vi "Simulation.vi"() -> ()   [LabVIEW 2013]
uses:
  <vilib>/Platform/TimedLoop/XDataNode/timing_clust.ctl
  <vilib>/Platform/TimedLoop/XDataNode/nitl_modes.ctl
  <vilib>/Platform/TimedLoop/XDataNode/wakeup.ctl
  <vilib>/Analysis/coordinate.llb/Angle Units.ctl
  <vilib>/Analysis/coordinate.llb/Angle Range (Degree).ctl
  <vilib>/Analysis/coordinate.llb/Wrap Angle (scalar).vi
  <vilib>/Utility/inputDevices.llb/closeJoystick.vi
  <vilib>/Utility/inputDevices.llb/joystickAcquire.vi
  <vilib>/Platform/TimedLoop/XDataNode/XDataNode.xnode
  <vilib>/Platform/TimedLoop/XDataNode/XDNodeRunTimeDep.lvlib
  Helper Functions/ProcessorHelperFunctions.lvlib
  <vilib>/Analysis/NI_AAL_Angle.lvlib
panel:
  in  "PID Gains":cluster{"P":dbl, "I":dbl, "D":dbl}={"P"=1.0, "I"=0.0, "D"=0.0}
  in  "Error Correction Speed":dbl=0.03
  out "Wheel Pos/Speed":picture
  out "Simulation Wheel Angles":dbl[](array[numeric])
  in  "Manual Motor Control":bool=TRUE
  in  "Motor Number":u8
  out "T1":dbl
  out "T3":dbl
  out "T2":dbl
  out "T4":dbl
  out "Wheel Target Angles":dbl[](array[numeric])
  out "Motor Output Values":u16[](array[slide]) scale=0.0..512.0
  out "Status LED":bool
  in  "stop":bool
  in  "ESTOP":bool
  out "TX Data":T1
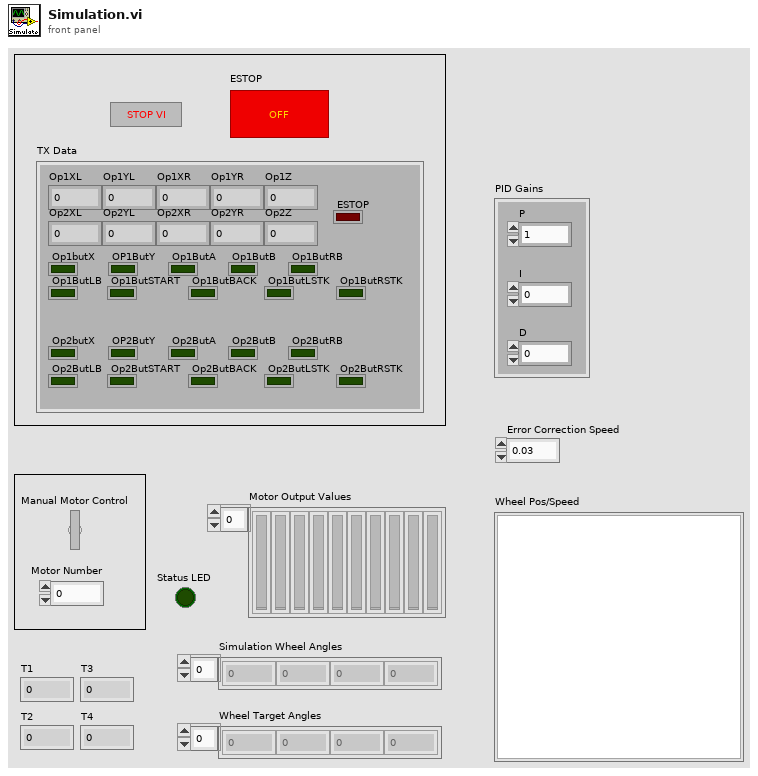
[diagram p1: front panel]
types:
  T1 = cluster{"Op2ButLSTK":bool, "Op2ButRSTK":bool, "Op1ButLSTK":bool, "Op1ButRSTK":bool, "Op1XL":i32, "Op1YL":i32, "Op1XR":i32, "Op1YR":i32, "Op1Z":i32, "Op2XL":i32, "Op2YL":i32, "Op2XR":i32, "Op2YR":i32, "Op2Z":i32, "ESTOP":bool, "Op1butX":bool, "OP1ButY":bool, "Op1ButA":bool, "Op1ButB":bool, "Op1ButRB":bool, "Op1ButLB":bool, "Op2butX":bool, "OP2ButY":bool, "Op2ButA":bool, "Op2ButB":bool, "Op2ButRB":bool, "Op2ButLB":bool, "Op2ButSTART":bool, "Op2ButBACK":bool, "Op1ButSTART":bool, "Op1ButBACK":bool}
  T2 = typedef "XDNodeRunTimeDep.lvlib/timing_clust.ctl" = cluster{"Expected End [f-1]":u64, "Actual End [f-1]":u64, "Finished Late? [f-1]":bool, "Expected End [i-1]":u64, "Actual End [i-1]":u64, "Finished Late? [i-1]":bool, "Expected Start [i]":u64, "Actual Start [i]":u64, "Expected Start [f]":u64, "Actual Start [f]":u64, "Source Name":string, "Structure Name":string, "Period":i64, "Deadline":i64, "Offset":i64, "Start":i64, "Priority":i32, "Timeout":i32, "Mode":T3, "Wakeup Reason":T4, "Error":errorcluster, "Source Type":string, "Secondary Source Type":string, "Global End Time":u64, "Global Start Time":u64, "Frame Duration":u64, "Iteration Duration":u64, "Assigned CPU":i32, "I/O Scan Engine Mode":u32}
  T3 = typedef "XDNodeRunTimeDep.lvlib/nitl_modes.ctl" = enum32{"No Change", "Process missed periods, maintain original phase", "Discard missed periods, maintain original phase", "Process missed periods, ignore original phase", "Discard missed periods, ignore original phase"}
  T4 = typedef "XDNodeRunTimeDep.lvlib/wakeup.ctl" = enum32{"Normal", "Aborted", "Asynchronous wakeup", "Timing source error", "Timed loop error", "Timeout"}
  T5 = typedef "NI_AAL_Angle.lvlib/Angle Range (Degree).ctl" = u16
  T6 = typedef "NI_AAL_Angle.lvlib/Angle Units.ctl" = i32
  T7 = cluster{"[0]":u16, "[1]":u16, "[2]":u16, "[3]":u16}
  T8 = cluster{"[0]":dbl, "[1]":dbl, "[2]":dbl, "[3]":dbl, "[4]":dbl, "[5]":dbl, "[6]":dbl, "[7]":dbl, "[8]":dbl}
  T9 = cluster{"Target Angles[0]":dbl, "Target Angles[1]":dbl, "Target Angles[2]":dbl, "Target Angles[3]":dbl}
  T10 = cluster{"X axis":i32, "Y axis":i32, "Z axis":i32, "X axis rotation":i32, "Y axis rotation":i32, "Z axis rotation":i32, "U axis":i32, "V axis":i32}
  T11 = cluster{"button 1":bool, "button 2":bool, "button 3":bool, "button 4":bool, "button 5":bool, "button 6":bool, "button 7":bool, "button 8":bool, "button 9":bool, "button 10":bool, "button 11":bool, "button 12":bool, "button 13":bool, "button 14":bool, "button 15":bool, "button 16":bool, "button 17":bool, "button 18":bool, "button 19":bool, "button 20":bool, "button 21":bool, "button 22":bool, "button 23":bool, "button 24":bool, "button 25":bool, "button 26":bool, "button 27":bool, "button 28":bool, "button 29":bool, "button 30":bool, "button 31":bool, "button 32":bool}
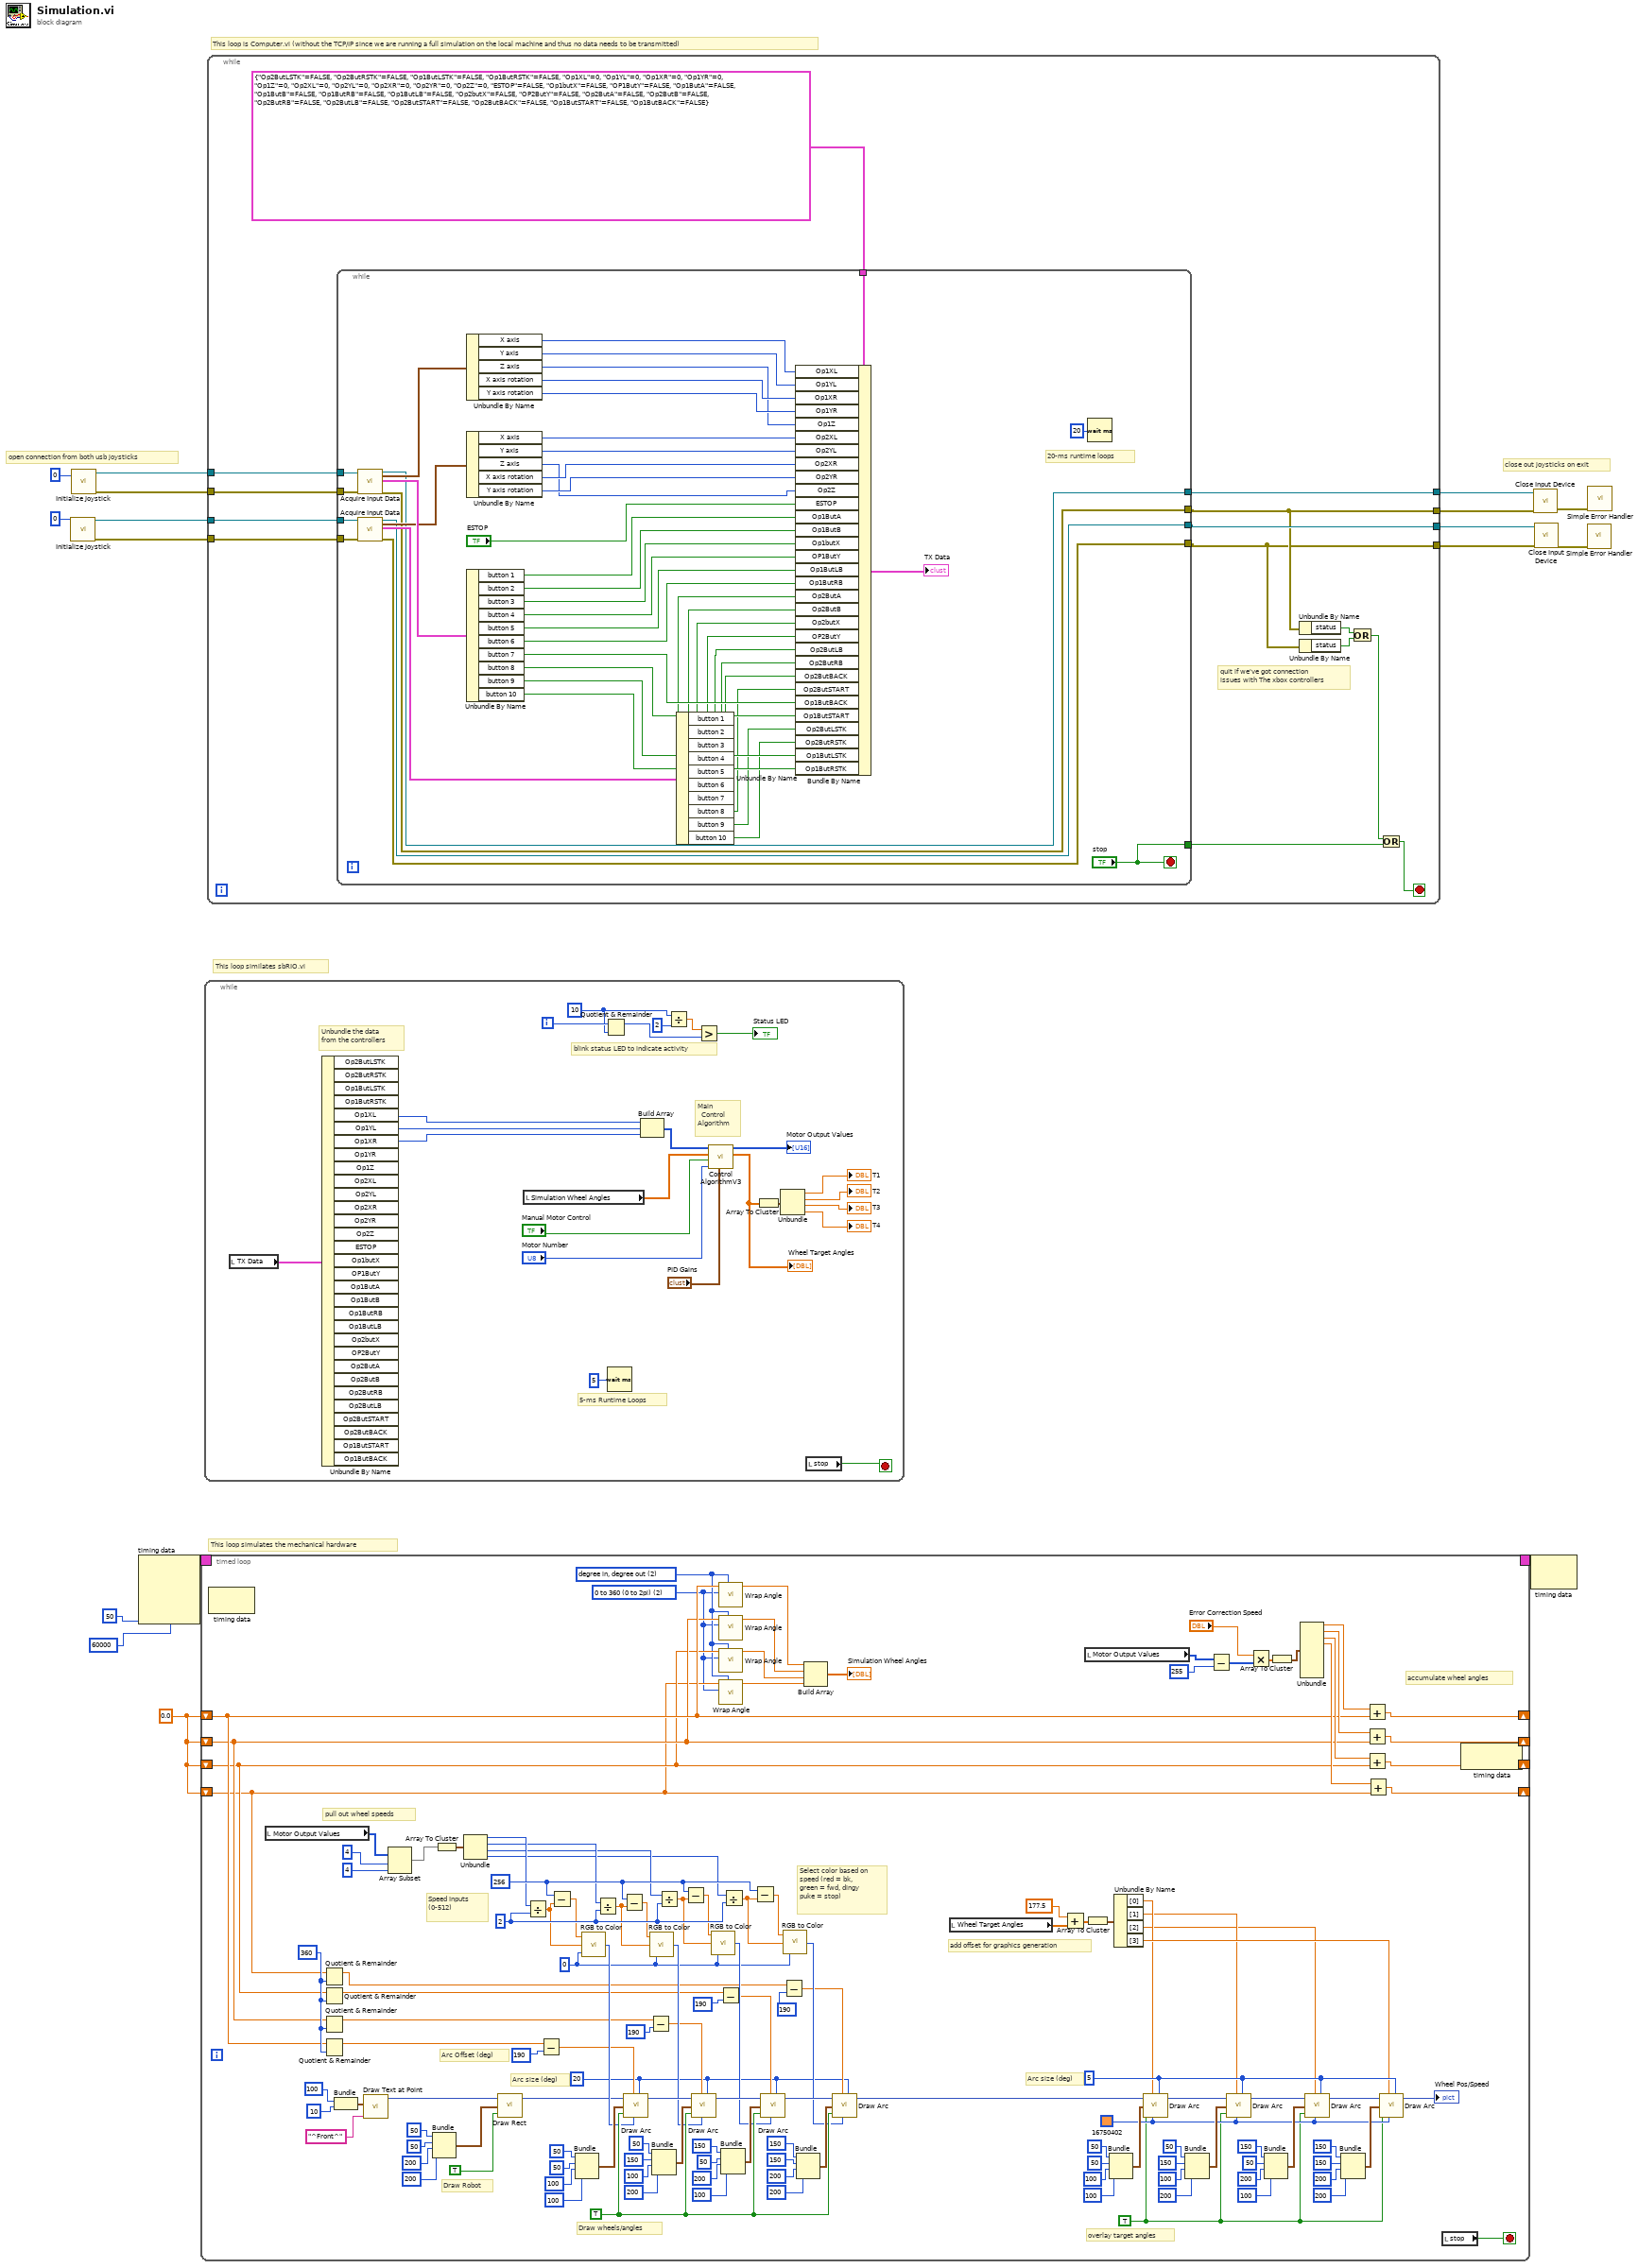
[diagram p0: block diagram]
diagram:
  w1 = 0.0
  # "This loop simulates the mechanical hardware"
  # "This loop similates sbRIO.vi"
  # "This loop is Computer.vi (without the TCP/IP since we are running a full simulation on the local machine and thus no data needs to be transmitted)"
  # "open connection from both usb joysticks"
  # "close out joysticks on exit"
  n1 = call <vilib>:"Initialize Joystick.vi"("device index"=0) -> ("error out"=w6:errorcluster, "device ID"=w7:refnum<k1>)  [unwired: 9 in]
  n2 = call <vilib>:"Initialize Joystick.vi"("device index"=0) -> ("error out"=w8:errorcluster, "device ID"=w9:refnum<k1>)  [unwired: 9 in]
  n3 = node-c288(50, 60000) -> (w5:T2)  [unwired: 2 in]
  n4 = timed-loop {
    timing: w5 -> [_]
    timing-out: [_] -> w4
    shift-right: [w148] -> _
    shift-left: w1 -> [w26]
    shift-right: [w147] -> _
    shift-left: w1 -> [w25]
    shift-right: [w149] -> _
    shift-left: w1 -> [w27]
    shift-right: [w150] -> _
    shift-left: w1 -> [w28]
    stop <- w31 stop-if-true
    w18 = T5 2 items=["none", "-180 to 180 (-pi to pi)", "0 to 360 (0 to 2pi)"] ("angle range")
    w19 = T6 2 items=["radian in, radian out", "radian in, degree out", "degree in, degree out", "degree in, radian out"] ("angle units")
    w33 = 360
    w53 = TRUE
    w56 = 5
    w57 = u32 16750402
    w87 = 20
    w32 = 0
    w104 = 2
    w105 = 256
    w117 = TRUE
    # "add offset for graphics generation"
    # "pull out wheel speeds"
    # "Arc size (deg)"
    # "overlay target angles"
    # "Arc Offset (deg)"
    # "Arc size (deg)"
    # "Speed Inputs (0-512)"
    # "Draw wheels/angles"
    # "Select color based on speed (red = bk, green = fwd, dingy puke = stop)"
    # "Draw Robot"
    # "accumulate wheel angles"
    n5 = node-c288() -> ()  [unwired: 1 in, 1 out]
    n6 = local read "Motor Output Values"() -> (w44:u16[])
    n7 = Quotient & Remainder(x=w25, y=w33) -> (x-y*floor(x/y)=w37:dbl)  [unwired: 1 out]
    n8 = Quotient & Remainder(x=w26, y=w33) -> (x-y*floor(x/y)=w36:dbl)  [unwired: 1 out]
    n9 = Quotient & Remainder(x=w27, y=w33) -> (x-y*floor(x/y)=w35:dbl)  [unwired: 1 out]
    n10 = Quotient & Remainder(x=w28, y=w33) -> (x-y*floor(x/y)=w34:dbl)  [unwired: 1 out]
    n11 = Bundle(100, 10) -> (w82:cluster{i32, i32})  [unwired: 1 in]
    n12 = call <vilib>:"Draw Text at Point.vi"("text"="^Front^", "origin"=w82) -> ("new picture"=w86:picture)  [unwired: 8 in, 1 out]
    n13 = Array Subset(array=w44, index=4, length=4) -> (w49:u16[])
    n14 = Bundle(50, 50, 200, 200) -> (w108:cluster{i32, i32, i32, i32})  [unwired: 1 in]
    n15 = Array To Cluster(array=w49) -> (cluster=w50:T7)
    n16 = Unbundle(w50) -> ("[0]"=w48:u16, "[1]"=w47:u16, "[2]"=w46:u16, "[3]"=w45:u16)
    n17 = call <vilib>:"Draw Rect.vi"("picture"=w86, "rect"=w108, "fill?(F)"=TRUE) -> ("new picture"=w106:picture)  [unwired: 6 in]
    n18 = Divide(x=w48, y=w104) -> (x/y=w103:dbl)
    n19 = Subtract(x=w34, y=190) -> (x-y=w94:dbl)
    n20 = Subtract(x=w105, y=w103) -> (x-y=w100:dbl)
    n21 = Bundle(50, 50, 100, 100) -> (w134:cluster{i32, i32, i32, i32})  [unwired: 1 in]
    n22 = call <vilib>:"RGB to Color.vi"("B"=w32, "G"=w103, "R"=w100) -> ("Color"=w116:u32)
    n23 = Divide(x=w47, y=w104) -> (x/y=w102:dbl)
    n24 = Subtract(x=w105, y=w102) -> (x-y=w99:dbl)
    n25 = call <vilib>:"Draw Arc.vi"("picture"=w106, "start angle[degrees]"=w94, "rect"=w134, "fill?(F)"=w117, "color(black)"=w116, "arc size[degrees]"=w87) -> ("new picture"=w140:picture)  [unwired: 3 in]
    n26 = Subtract(x=w35, y=190) -> (x-y=w90:dbl)
    n27 = call <vilib>:"RGB to Color.vi"("B"=w32, "G"=w102, "R"=w99) -> ("Color"=w115:u32)
    n28 = Bundle(50, 150, 100, 200) -> (w120:cluster{i32, i32, i32, i32})  [unwired: 1 in]
    n29 = Divide(x=w46, y=w104) -> (x/y=w98:dbl)
    n30 = Subtract(x=w105, y=w98) -> (x-y=w97:dbl)
    n31 = call <vilib>:"Draw Arc.vi"("picture"=w140, "start angle[degrees]"=w90, "rect"=w120, "fill?(F)"=w117, "color(black)"=w115, "arc size[degrees]"=w87) -> ("new picture"=w139:picture)  [unwired: 3 in]
    n32 = call <vilib>:"RGB to Color.vi"("B"=w32, "G"=w98, "R"=w97) -> ("Color"=w114:u32)
    n33 = call-poly <vilib>:"Wrap Angle.vi"("angle units"=w19, "angle range"=w18, "angle in"=w28) -> ("angle out"=w24:dbl)  [unwired: 7 in, 1 out]
    n34 = call-poly <vilib>:"Wrap Angle.vi"("angle units"=w19, "angle range"=w18, "angle in"=w27) -> ("angle out"=w23:dbl)  [unwired: 7 in, 1 out]
    n35 = call-poly <vilib>:"Wrap Angle.vi"("angle units"=w19, "angle range"=w18, "angle in"=w26) -> ("angle out"=w22:dbl)  [unwired: 7 in, 1 out]
    n36 = call-poly <vilib>:"Wrap Angle.vi"("angle units"=w19, "angle range"=w18, "angle in"=w25) -> ("angle out"=w21:dbl)  [unwired: 7 in, 1 out]
    n37 = Subtract(x=w36, y=190) -> (x-y=w89:dbl)
    n38 = Bundle(150, 50, 200, 100) -> (w119:cluster{i32, i32, i32, i32})  [unwired: 1 in]
    n39 = Divide(x=w45, y=w104) -> (x/y=w101:dbl)
    n40 = Subtract(x=w105, y=w101) -> (x-y=w96:dbl)
    n41 = call <vilib>:"Draw Arc.vi"("picture"=w139, "start angle[degrees]"=w89, "rect"=w119, "fill?(F)"=w117, "color(black)"=w114, "arc size[degrees]"=w87) -> ("new picture"=w138:picture)  [unwired: 3 in]
    n42 = Subtract(x=w37, y=190) -> (x-y=w88:dbl)
    n43 = call <vilib>:"RGB to Color.vi"("B"=w32, "G"=w101, "R"=w96) -> ("Color"=w113:u32)
    n44 = Bundle(150, 150, 200, 200) -> (w118:cluster{i32, i32, i32, i32})  [unwired: 1 in]
    n45 = Build Array(w24, w23, w22, w21) -> (→"Simulation Wheel Angles":dbl[])
    n46 = call <vilib>:"Draw Arc.vi"("picture"=w138, "start angle[degrees]"=w88, "rect"=w118, "fill?(F)"=w117, "color(black)"=w113, "arc size[degrees]"=w87) -> ("new picture"=w81:picture)  [unwired: 3 in]
    n47 = local read "Wheel Target Angles"() -> (w43:dbl[])
    n48 = Add(x=177.5, y=w43) -> (x+y=w42:dbl[])
    n49 = local read "Motor Output Values"() -> (w29:u16[])
    n50 = Array To Cluster(array=w42) -> (cluster=w55:T8)
    n51 = Bundle(50, 50, 100, 100) -> (w75:cluster{i32, i32, i32, i32})  [unwired: 1 in]
    n52 = Unbundle By Name(w55) -> ("[0]"=w40:dbl, "[1]"=w39:dbl, "[2]"=w38:dbl, "[3]"=w54:dbl)
    n53 = call <vilib>:"Draw Arc.vi"("picture"=w81, "start angle[degrees]"=w40, "rect"=w75, "fill?(F)"=w53, "color(black)"=w57, "arc size[degrees]"=w56) -> ("new picture"=w80:picture)  [unwired: 3 in]
    n54 = Bundle(50, 150, 100, 200) -> (w69:cluster{i32, i32, i32, i32})  [unwired: 1 in]
    n55 = Subtract(x=w29, y=255) -> (x-y=w152:i32[])
    n56 = call <vilib>:"Draw Arc.vi"("picture"=w80, "start angle[degrees]"=w39, "rect"=w69, "fill?(F)"=w53, "color(black)"=w57, "arc size[degrees]"=w56) -> ("new picture"=w63:picture)  [unwired: 3 in]
    n57 = Multiply(x="Error Correction Speed", y=w152) -> (x*y=w146:dbl[])
    n58 = Bundle(150, 50, 200, 100) -> (w64:cluster{i32, i32, i32, i32})  [unwired: 1 in]
    n59 = Array To Cluster(array=w146) -> (cluster=w151:T8)
    n60 = Unbundle(w151) -> ("[0]"=w144:dbl, "[1]"=w143:dbl, "[2]"=w142:dbl, "[3]"=w141:dbl)  [unwired: 5 out]
    n61 = call <vilib>:"Draw Arc.vi"("picture"=w63, "start angle[degrees]"=w38, "rect"=w64, "fill?(F)"=w53, "color(black)"=w57, "arc size[degrees]"=w56) -> ("new picture"=w79:picture)  [unwired: 3 in]
    n62 = Bundle(150, 150, 200, 200) -> (w58:cluster{i32, i32, i32, i32})  [unwired: 1 in]
    n63 = Add(x=w144, y=w28) -> (x+y=w150:dbl)
    n64 = Add(x=w143, y=w27) -> (x+y=w149:dbl)
    n65 = Add(x=w142, y=w26) -> (x+y=w148:dbl)
    n66 = Add(x=w141, y=w25) -> (x+y=w147:dbl)
    n67 = call <vilib>:"Draw Arc.vi"("picture"=w79, "start angle[degrees]"=w54, "rect"=w58, "fill?(F)"=w53, "color(black)"=w57, "arc size[degrees]"=w56) -> ("new picture"=→"Wheel Pos/Speed":picture)  [unwired: 3 in]
    n68 = local read "stop"() -> (w31:bool)
    n69 = node-c288() -> ()  [unwired: 1 in, 1 out]
  }
  n70 = while {
    i -> [w178]
    stop <- w163 stop-if-true
    w174 = 10
    # "Unbundle the data\nfrom the controllers"
    # "Main\n  Control\nAlgorithm"
    # "blink status LED to indicate activity"
    # "5-ms Runtime Loops"
    n71 = local read "TX Data"() -> (w165:T1)
    n72 = Unbundle By Name(w165) -> ("Op1XL"=w168:i32, "Op1YL"=w167:i32, "Op1XR"=w166:i32)  [unwired: 28 out]
    n73 = local read "Simulation Wheel Angles"() -> (w161:dbl[])
    n74 = Quotient & Remainder(x=w178, y=w174) -> (x-y*floor(x/y)=w176:i32)  [unwired: 1 out]
    n75 = Wait (ms)(milliseconds to wait=u32 5) -> ()  [unwired: 1 out]
    n76 = Build Array(w168, w167, w166) -> (w162:i32[])
    n77 = Divide(x=w174, y=2) -> (x/y=w175:dbl)
    n78 = Greater?(x=w175, y=w176) -> (0:→"Status LED":bool)
    n79 = call "Control AlgorithmV3.vi"("PID Gains"="PID Gains", "Motor to Control"="Motor Number", "Manual Control"="Manual Motor Control", "Wheel Angles"=w161, "JoystickIn"=w162) -> ("Target Angles"=w157:dbl[], "MotorsOut"=→"Motor Output Values":u16[])  [unwired: 5 in]
    "Wheel Target Angles" <- w157
    n80 = Array To Cluster(array=w157) -> (cluster=w173:T9)
    n81 = Unbundle(w173) -> ("Target Angles[0]"=→"T1":dbl, "Target Angles[1]"=→"T2":dbl, "Target Angles[2]"=→"T3":dbl, "Target Angles[3]"=→"T4":dbl)
    n82 = local read "stop"() -> (w163:bool)
  }
  n83 = while {
    tunnel: [w192] -> w15
    tunnel: [w190] -> w14
    tunnel: [w191] -> w13
    tunnel: [w189] -> w12
    tunnel: w9 -> [w185]
    tunnel: w8 -> [w184]
    tunnel: w7 -> [w183]
    tunnel: w6 -> [w182]
    stop <- w186 stop-if-true
    # "quit if we've got connection \nissues with The xbox controllers"
    n84 = while {
      tunnel: w185 -> [w239]
      tunnel: w184 -> [w238]
      tunnel: T1 {"Op2ButLSTK"=FALSE, "Op2ButRSTK"=FALSE, "Op1ButLSTK"=FALSE, "Op1ButRSTK"=FALSE, "Op1XL"=0, "Op1YL"=0, "Op1XR"=0, "Op1YR"=0, "Op1Z"=0, "Op2XL"=0, "Op2YL"=0, "Op2XR"=0, "Op2YR"=0, "Op2Z"=0, "ESTOP"=FALSE, "Op1butX"=FALSE, "OP1ButY"=FALSE, "Op1ButA"=FALSE, "Op1ButB"=FALSE, "Op1ButRB"=FALSE, "Op1ButLB"=FALSE, "Op2butX"=FALSE, "OP2ButY"=FALSE, "Op2ButA"=FALSE, "Op2ButB"=FALSE, "Op2ButRB"=FALSE, "Op2ButLB"=FALSE, "Op2ButSTART"=FALSE, "Op2ButBACK"=FALSE, "Op1ButSTART"=FALSE, "Op1ButBACK"=FALSE} -> [w237]
      tunnel: w183 -> [w200]
      tunnel: w182 -> [w199]
      tunnel: [w198] -> w192
      tunnel: [w197] -> w191
      tunnel: [w196] -> w190
      tunnel: [w195] -> w189
      tunnel: ["stop"] -> w181
      stop <- "stop" stop-if-true
      # "20-ms runtime loops"
      n85 = call-poly <vilib>:"Acquire Input Data.vi"("device ID"=w239, "error in (no error)"=w238) -> ("device ID"=w198:refnum<k1>, "axis info"=w220:T10, "button info"=w219:T11, "error out"=w196:errorcluster)  [unwired: 13 in, 1 out]
      n86 = call-poly <vilib>:"Acquire Input Data.vi"("device ID"=w200, "error in (no error)"=w199) -> ("device ID"=w197:refnum<k1>, "axis info"=w201:T10, "button info"=w202:T11, "error out"=w195:errorcluster)  [unwired: 13 in, 1 out]
      n87 = Unbundle By Name(w220) -> ("X axis"=w234:i32, "Y axis"=w233:i32, "Z axis"=w204:i32, "X axis rotation"=w232:i32, "Y axis rotation"=w231:i32)
      n88 = Unbundle By Name(w201) -> ("X axis"=w218:i32, "Y axis"=w217:i32, "Z axis"=w203:i32, "X axis rotation"=w216:i32, "Y axis rotation"=w215:i32)
      n89 = Unbundle By Name(w219) -> ("button 1"=w230:bool, "button 2"=w229:bool, "button 3"=w228:bool, "button 4"=w227:bool, "button 5"=w226:bool, "button 6"=w225:bool, "button 7"=w224:bool, "button 8"=w223:bool, "button 9"=w222:bool, "button 10"=w221:bool)
      n90 = Unbundle By Name(w202) -> ("button 1"=w214:bool, "button 2"=w213:bool, "button 3"=w212:bool, "button 4"=w211:bool, "button 5"=w210:bool, "button 6"=w209:bool, "button 7"=w208:bool, "button 8"=w207:bool, "button 9"=w206:bool, "button 10"=w205:bool)
      n91 = Bundle By Name(cluster=w237, "Op1XL"=w234, "Op1YL"=w233, "Op1XR"=w232, "Op1YR"=w231, "Op1Z"=w204, "Op2XL"=w218, "Op2YL"=w217, "Op2XR"=w216, "Op2YR"=w215, "Op2Z"=w203, "ESTOP"="ESTOP", "Op1ButA"=w230, "Op1ButB"=w229, "Op1butX"=w228, "OP1ButY"=w227, "Op1ButLB"=w226, "Op1ButRB"=w225, "Op2ButA"=w214, "Op2ButB"=w213, "Op2butX"=w212, "OP2ButY"=w211, "Op2ButLB"=w210, "Op2ButRB"=w209, "Op2ButBACK"=w208, "Op2ButSTART"=w207, "Op1ButBACK"=w224, "Op1ButSTART"=w223, "Op2ButLSTK"=w206, "Op2ButRSTK"=w205, "Op1ButLSTK"=w222, "Op1ButRSTK"=w221) -> (→"TX Data":T1)
      n92 = Wait (ms)(milliseconds to wait=u32 20) -> ()  [unwired: 1 out]
    }
    n93 = Unbundle By Name(w190) -> ("status"=w188:bool)
    n94 = Unbundle By Name(w189) -> ("status"=w187:bool)
    n95 = Or(x=w188, y=w187) -> (x .or. y?=w180:bool)
    n96 = Or(x=w180, y=w181) -> (x .or. y?=w186:bool)
  }
  n97 = node-c288(w4) -> ()  [unwired: 1 out]
  n98 = call-poly <vilib>:"Close Input Device.vi"("error in (no error)"=w14, "device ID"=w15) -> ("error out"=w16:errorcluster)  [unwired: 8 in]
  n99 = call-poly <vilib>:"Close Input Device.vi"("error in (no error)"=w12, "device ID"=w13) -> ("error out"=w17:errorcluster)  [unwired: 8 in]
  n100 = call <vilib>:"Simple Error Handler.vi"("error in (no error)"=w17) -> ()  [unwired: 4 in, 5 out]
  n101 = call <vilib>:"Simple Error Handler.vi"("error in (no error)"=w16) -> ()  [unwired: 4 in, 5 out]
